vi "Write Rotation.vi"(8 "error in (no error)":errorcluster, 10 "Rotation":cluster{"Axis":T1, "Angle":sgl}, 11 "Velodyne 3D LIDAR in":refnum<class "Velodyne 3D LIDAR.lvclass">) -> (0 "error out":errorcluster, 3 "Velodyne 3D LIDAR out":refnum<class "Velodyne 3D LIDAR.lvclass">)   [LabVIEW 2017, in "NI_Robotics_Simulator.lvlib" / "Velodyne 3D LIDAR.lvclass"]
uses:
  <vilib>/robotics/Simulator/Plugin/Sensor/Velodyne 3D LIDAR/Velodyne 3D LIDAR.lvclass
  <vilib>/Utility/miscctls.llb/LV3DPointTypeDef.ctl
  <vilib>/robotics/Simulator/Plugin/Sensor/Velodyne 3D LIDAR/Velodyne 3D LIDAR.lvclass/Velodyne 3D LIDAR.ctl
  <vilib>/Analysis/baseanly.llb/Real A x B.vi
  <vilib>/robotics/Kinematics/Angle Vector to Rotation Matrix.vi
  <vilib>/Analysis/_algsub.llb/Vector Norm.vi
  <vilib>/Analysis/_algsub.llb/Real Vector Norm.vi
  <vilib>/Analysis/baseanly.llb/Outer Product.vi
  <vilib>/Analysis/baseanly.llb/Real Outer Product.vi
  <vilib>/robotics/Kinematics/Create Lie Group Matrix.vi
  <vilib>/robotics/Kinematics/Rotation Matrix to Angle Vector.vi
  <vilib>/Analysis/Matrix/Numeric/Add/Add.vi
  <vilib>/Analysis/Matrix/Numeric/Add/Add - RM,RM.vi
  <vilib>/Analysis/Matrix/Numeric/Multiply/Multiply.vi
  <vilib>/Analysis/Matrix/Numeric/Multiply/Multiply - R,RM.vi
  <vilib>/Analysis/Matrix/Numeric/Multiply/Multiply - RM,R.vi
  <vilib>/Analysis/7linalg.llb/Create Special Matrix.vi
  <vilib>/Analysis/7linalg.llb/Create Special Real Matrix.vi
  <vilib>/robotics/Simulator/Robot Factory/Sensor/Base/ODESimulator_Base_Sensor.lvclass
  <vilib>/robotics/Simulator/3D-Physics/Sphere/3D_Physics_Sphere.lvclass
  <vilib>/robotics/Simulator/Robot Factory/Sensor/LIDAR/ODESimulator_LIDAR.lvclass
  <vilib>/robotics/Simulator/NI_Robotics_Simulator.lvlib
  <vilib>/Analysis/NI_AALBase.lvlib
  <vilib>/robotics/Simulator/Robot Factory/Joint/ODESimulator_Joint.lvclass
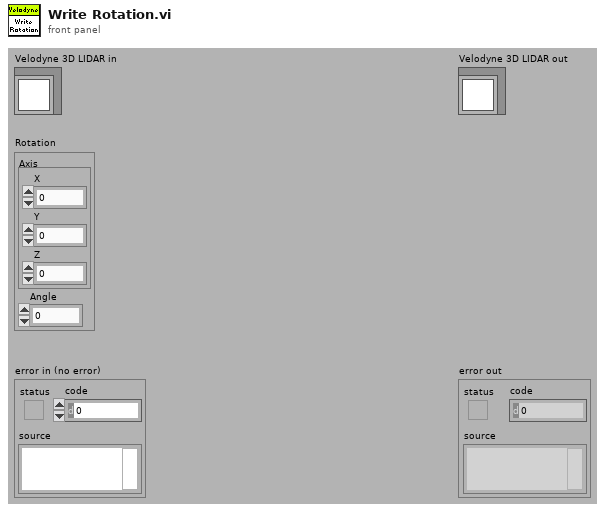
[diagram p1: front panel]
types:
  T1 = typedef "LV3DPointTypeDef.ctl" = cluster{"X":sgl, "Y":sgl, "Z":sgl}
  T2 = typedef "NI_Matrix.lvlib/RealMatrix.ctl" = dbl[][]
  T3 = cluster{"Axis":cluster{"X":dbl, "Y":dbl, "Z":dbl}, "Angle":dbl}
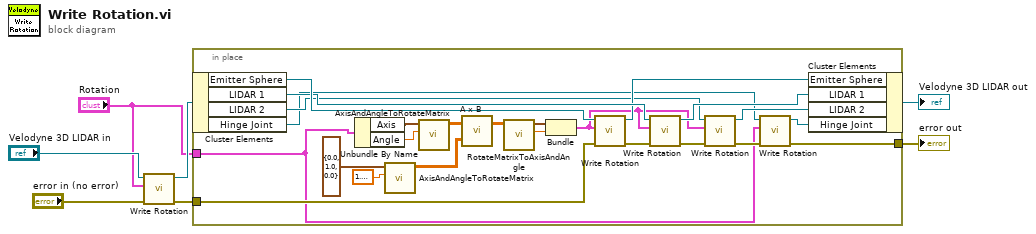
[diagram p0: block diagram]
diagram:
  n1 = call-parent <vilib>:"Write Rotation.vi"("error in (no error)"="error in (no error)", "Rotation"="Rotation", "ODESimulator_Base_Sensor in"="Velodyne 3D LIDAR in") -> ("error out"=w2:errorcluster, "ODESimulator_Base_Sensor out"=w5:refnum<class "Velodyne 3D LIDAR.lvclass">)  [unwired: 7 in]
  n2 = in-place {
    in-place-border: "Rotation" -> [w8]
    in-place-border: w2 -> [w10]
    in-place-border: [w9] -> w1
    n3 = in-place-cluster #1(w5) -> ("Emitter Sphere"=w24:refnum<class "3D_Physics_Sphere.lvclass">, "LIDAR 1"=w21:refnum<class "ODESimulator_LIDAR.lvclass">, "LIDAR 2"=w17:refnum<class "ODESimulator_LIDAR.lvclass">, "Hinge Joint"=w14:refnum<class "ODESimulator_Joint.lvclass">)
    n4 = Unbundle By Name(w8) -> ("Axis"=w31:T1, "Angle"=w30:sgl)
    n5 = call <vilib>:"AxisAndAngleToRotateMatrix.vi"("Angle"=1.5707963267948966, "Axis"=T1 {"X"=0.0, "Y"=1.0, "Z"=0.0}) -> ("Rotation Matrix"=w26:dbl[][])  [unwired: 8 in, 1 out]
    n6 = call <vilib>:"AxisAndAngleToRotateMatrix.vi"("Angle"=w30, "Axis"=w31) -> ("Rotation Matrix"=w27:dbl[][])  [unwired: 8 in, 1 out]
    n7 = call-poly <vilib>:"A x B.vi"("B"=w26, "A"=w27) -> ("A x B"=w25:T2)  [unwired: 1 out]
    n8 = call <vilib>:"RotateMatrixToAxisAndAngle.vi"("Rotation Matrix"=w25) -> ("Angle"=w23:dbl, "Axis"=w22:cluster{"X":dbl, "Y":dbl, "Z":dbl})  [unwired: 8 in, 1 out]
    n9 = Bundle("Axis"=w22, "Angle"=w23) -> (w13:T3)  [unwired: 1 in]
    n10 = call-dynamic <vilib>:"Write Rotation.vi"("error in (no error)"=w10, "Rotation"=w13, "Base in"=w24) -> ("error out"=w15:errorcluster, "Base out"=w20:refnum<class "3D_Physics_Sphere.lvclass">)  [unwired: 7 in]
    n11 = call-dynamic <vilib>:"Write Rotation.vi"("error in (no error)"=w15, "Rotation"=w13, "ODESimulator_Base_Sensor in"=w21) -> ("error out"=w19:errorcluster, "ODESimulator_Base_Sensor out"=w18:refnum<class "ODESimulator_LIDAR.lvclass">)  [unwired: 7 in]
    n12 = call-dynamic <vilib>:"Write Rotation.vi"("error in (no error)"=w19, "Rotation"=w13, "ODESimulator_Base_Sensor in"=w17) -> ("error out"=w12:errorcluster, "ODESimulator_Base_Sensor out"=w16:refnum<class "ODESimulator_LIDAR.lvclass">)  [unwired: 7 in]
    n13 = call <vilib>:"Write Rotation.vi"("error in (no error)"=w12, "Rotation"=w8, "ODESimulator_Joint in"=w14) -> ("error out"=w9:errorcluster, "ODESimulator_Joint out"=w11:refnum<class "ODESimulator_Joint.lvclass">)  [unwired: 7 in]
    n14 = in-place-cluster #1("Emitter Sphere"=w20, "LIDAR 1"=w18, "LIDAR 2"=w16, "Hinge Joint"=w11) -> (→"Velodyne 3D LIDAR out":refnum<class "Velodyne 3D LIDAR.lvclass">)
  }
  "error out" <- w1
